vi "DataXML addParameter.vi"(5 "param name":string, 7 "param value":string, 8 "error in (no error)":errorcluster, 10 "tag node in":refnum<k20>, 11 "DataXML in":refnum<class "DataXML.lvclass">) -> (0 "error out":errorcluster, 2 "tag node out":refnum<k20>, 3 "DataXML out":refnum<class "DataXML.lvclass">)   [LabVIEW 2018, in "DataXML.lvclass"]
uses:
  DataXML.lvclass
  DataXML.lvclass/DataXML.ctl
  <vilib>/xml/Close Reference(Node).vi
  <resource>/objmgr/DOMUserDefRef.rc
  <vilib>/xml/NI_XML.lvlib
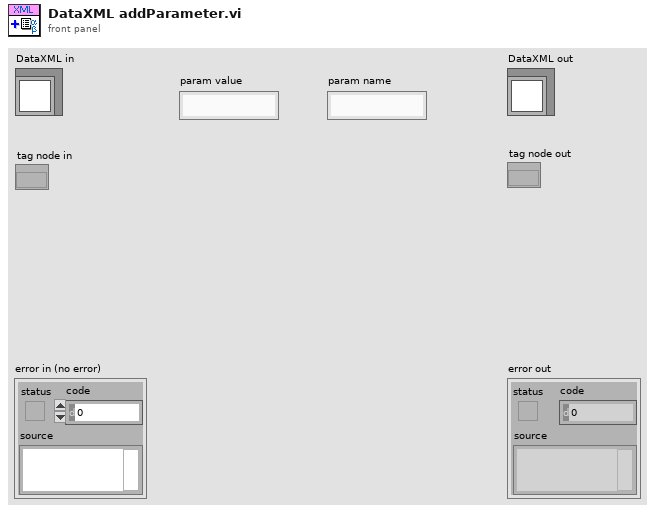
[diagram p1: front panel]
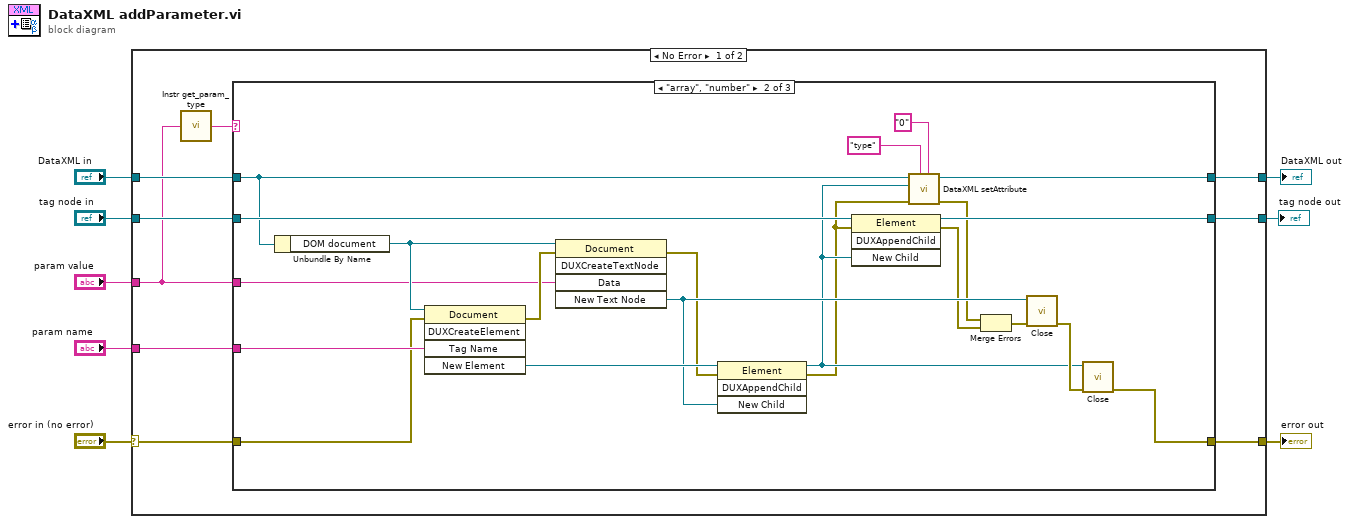
[diagram p0: block diagram]
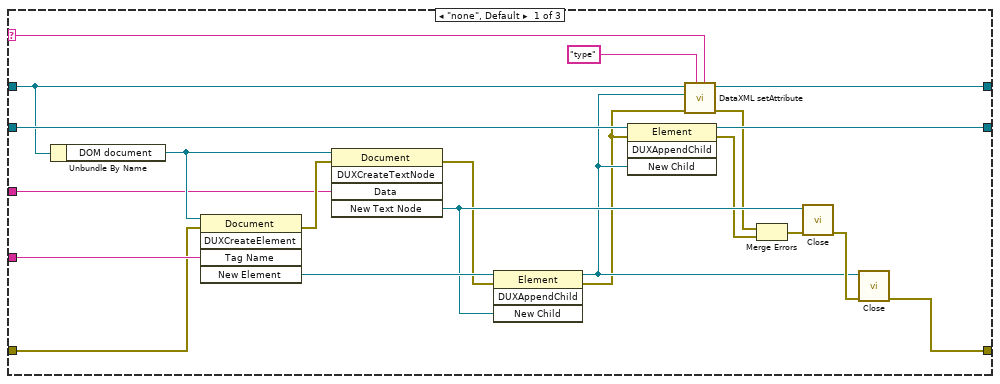
[diagram p2: hidden frame]
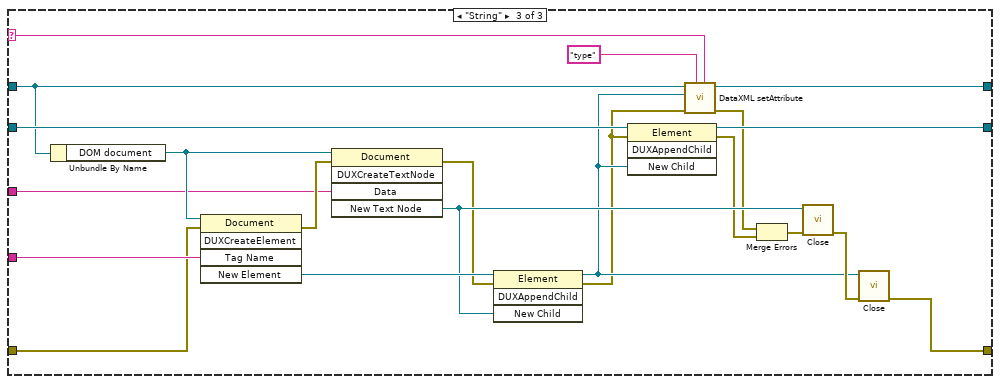
[diagram p3: hidden frame]
diagram:
  n1 = case shown="No Error" "error in (no error)" {
    selector: "error in (no error)" -> [w16 w82]
    tunnel: [w13 w82] -> w7
    tunnel: [w11 w81] -> w5
    tunnel: "DataXML in" -> [w12 w81]
    tunnel: "param name" -> [w17 _]
    tunnel: "param value" -> [w10 _]
    tunnel: "tag node in" -> [w15 _]
    tunnel: [w14 _] -> w1
    frame No Error {
      n2 = call "Instr get_param_type.vi"("value_array"=w10) -> ("type"=w9:string)
      n3 = case shown="\"array\", \"number\"" w9 {
        selector: w9 -> [w18 _ w60]
        tunnel: w17 -> [w37 w58 w79]
        tunnel: w16 -> [w34 w55 w76]
        tunnel: w15 -> [w33 w54 w75]
        tunnel: [w30 w51 w72] -> w14
        tunnel: [w29 w50 w71] -> w13
        tunnel: w12 -> [w27 w48 w69]
        tunnel: [w26 w47 w68] -> w11
        tunnel: w10 -> [w19 w40 w61]
        frame "none", Default {
          n4 = Unbundle By Name(w27) -> ("DOM document"=w35:refnum<k20>)
          n5 = invoke class="Document" method="DUXCreateElement"(reference=w35, error in=w34, "Tag Name"=w37) -> (error out=w38:errorcluster, "New Element"=w36:refnum<k20>)  [unwired: 2 in, 3 out]
          n6 = invoke class="Document" method="DUXCreateTextNode"(reference=w35, error in=w38, "Data"=w19) -> (error out=w28:errorcluster, "New Text Node"=w32:refnum<k20>)  [unwired: 2 in, 3 out]
          n7 = invoke class="Element" method="DUXAppendChild"(reference=w36, error in=w28, "New Child"=w32) -> (reference out=w24:refnum<k20>, error out=w23:errorcluster)  [unwired: 1 in, 2 out]
          n8 = invoke class="Element" method="DUXAppendChild"(reference=w33, error in=w23, "New Child"=w24) -> (reference out=w30:refnum<k20>, error out=w21:errorcluster)  [unwired: 1 in, 2 out]
          n9 = call "DataXML setAttribute.vi"("attr_value"=w18, "attr_name"="type", "error in (no error)"=w23, "target node in"=w24, "DataXML in"=w27) -> ("error out"=w22:errorcluster, "DataXML out"=w26:refnum<class "DataXML.lvclass">)  [unwired: 4 in, 1 out]
          n10 = Merge Errors(w22, w21) -> (w20:errorcluster)
          n11 = call-poly <vilib>:"Close.vi"("error in (no error)"=w20, "node"=w32) -> ("error out"=w31:errorcluster)  [unwired: 7 out]
          n12 = call-poly <vilib>:"Close.vi"("error in (no error)"=w31, "node"=w24) -> ("error out"=w29:errorcluster)  [unwired: 7 out]
        }
        frame "array", "number" {
          n13 = Unbundle By Name(w48) -> ("DOM document"=w56:refnum<k20>)
          n14 = invoke class="Document" method="DUXCreateElement"(reference=w56, error in=w55, "Tag Name"=w58) -> (error out=w59:errorcluster, "New Element"=w57:refnum<k20>)  [unwired: 2 in, 3 out]
          n15 = invoke class="Document" method="DUXCreateTextNode"(reference=w56, error in=w59, "Data"=w40) -> (error out=w49:errorcluster, "New Text Node"=w53:refnum<k20>)  [unwired: 2 in, 3 out]
          n16 = invoke class="Element" method="DUXAppendChild"(reference=w57, error in=w49, "New Child"=w53) -> (reference out=w45:refnum<k20>, error out=w44:errorcluster)  [unwired: 1 in, 2 out]
          n17 = invoke class="Element" method="DUXAppendChild"(reference=w54, error in=w44, "New Child"=w45) -> (reference out=w51:refnum<k20>, error out=w42:errorcluster)  [unwired: 1 in, 2 out]
          n18 = call "DataXML setAttribute.vi"("attr_value"="0", "attr_name"="type", "error in (no error)"=w44, "target node in"=w45, "DataXML in"=w48) -> ("error out"=w43:errorcluster, "DataXML out"=w47:refnum<class "DataXML.lvclass">)  [unwired: 4 in, 1 out]
          n19 = Merge Errors(w43, w42) -> (w41:errorcluster)
          n20 = call-poly <vilib>:"Close.vi"("error in (no error)"=w41, "node"=w53) -> ("error out"=w52:errorcluster)  [unwired: 7 out]
          n21 = call-poly <vilib>:"Close.vi"("error in (no error)"=w52, "node"=w45) -> ("error out"=w50:errorcluster)  [unwired: 7 out]
        }
        frame "String" {
          n22 = Unbundle By Name(w69) -> ("DOM document"=w77:refnum<k20>)
          n23 = invoke class="Document" method="DUXCreateElement"(reference=w77, error in=w76, "Tag Name"=w79) -> (error out=w80:errorcluster, "New Element"=w78:refnum<k20>)  [unwired: 2 in, 3 out]
          n24 = invoke class="Document" method="DUXCreateTextNode"(reference=w77, error in=w80, "Data"=w61) -> (error out=w70:errorcluster, "New Text Node"=w74:refnum<k20>)  [unwired: 2 in, 3 out]
          n25 = invoke class="Element" method="DUXAppendChild"(reference=w78, error in=w70, "New Child"=w74) -> (reference out=w66:refnum<k20>, error out=w65:errorcluster)  [unwired: 1 in, 2 out]
          n26 = invoke class="Element" method="DUXAppendChild"(reference=w75, error in=w65, "New Child"=w66) -> (reference out=w72:refnum<k20>, error out=w63:errorcluster)  [unwired: 1 in, 2 out]
          n27 = call "DataXML setAttribute.vi"("attr_value"=w60, "attr_name"="type", "error in (no error)"=w65, "target node in"=w66, "DataXML in"=w69) -> ("error out"=w64:errorcluster, "DataXML out"=w68:refnum<class "DataXML.lvclass">)  [unwired: 4 in, 1 out]
          n28 = Merge Errors(w64, w63) -> (w62:errorcluster)
          n29 = call-poly <vilib>:"Close.vi"("error in (no error)"=w62, "node"=w74) -> ("error out"=w73:errorcluster)  [unwired: 7 out]
          n30 = call-poly <vilib>:"Close.vi"("error in (no error)"=w73, "node"=w66) -> ("error out"=w71:errorcluster)  [unwired: 7 out]
        }
      }
    }
    frame Error {
    }
  }
  "error out" <- w7
  "DataXML out" <- w5
  "tag node out" <- w1
